vi "Teleop.vi"(10 "Match Info":T1={"Autonomous Elapsed Seconds"=0.0, "TeleOp Elapsed Seconds"=0.0, "Disabled Elapsed Seconds"=0.0, "Visited Autonomous"=FALSE, "Visited TeleOp"=FALSE, "Visited Disabled"=FALSE, "Autonomous Settings"={"Autonomous Style"=enum."Independent", "VI Refnum"=refnum}}, 11 "Call Context":T2) -> ()   [LabVIEW 2014]
doc: "This VI is called for each TeleOp packet received from the DS where the robot is not disabled. It is often used to read from the joysticks and update I/O or to update setpoints for timed control loops. It should complete and return within 20 milliseconds or it may miss DS packets."
uses:
  <vilib>/Rock Robotics/WPI/DriverStation/WPI_DriverStationDerivedRobotMode.ctl
  <vilib>/Rock Robotics/WPI/DriverStation/WPI_DriverStationMatch Info.ctl
  Drivetrain Code/Drivetrain Control.ctl
  Drivetrain Code/Drivetrain Mode.ctl
  Common Code/Solenoid Command.ctl
  <vilib>/Rock Robotics/WPI/Joystick/WPI_JoystickGetSetRefNum.vi
  <vilib>/Rock Robotics/Network Tables/SD Write Boolean Array.vi
  <vilib>/Rock Robotics/Network Tables/SD Write Numeric Array.vi
  Robot Global Data.vi
  <vilib>/Rock Robotics/Network Tables/SD Read Number.vi
  <vilib>/Rock Robotics/WPI/Solenoid/WPI_SolenoidSetEnum.vi
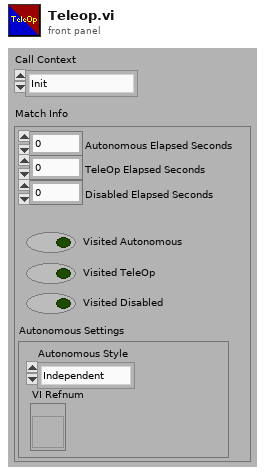
[diagram p1: front panel]
types:
  T1 = typedef "WPI_DriverStationMatch Info.ctl" = cluster{"Autonomous Elapsed Seconds":dbl, "TeleOp Elapsed Seconds":dbl, "Disabled Elapsed Seconds":dbl, "Visited Autonomous":bool, "Visited TeleOp":bool, "Visited Disabled":bool, "Autonomous Settings":cluster{"Autonomous Style":enum16{"Iterative", "Independent"}, "VI Refnum":refnum<vi>}}
  T2 = typedef "WPI_DriverStationDerivedRobotMode.ctl" = enum16{"Init", "Execute", "Stop"}
  T3 = typedef "Solenoid Command.ctl" = cluster{"Lift":bool, "Gripper":bool}
  T4 = typedef "Drivetrain Control.ctl" = cluster{"Mode":T5, "X":dbl, "Y":dbl, "Heading Target":dbl, "Y Target":dbl}
  T5 = typedef "Drivetrain Mode.ctl" = enum16{"Manual", "Gyro Steer", "Vision Steer", "Drive Distance"}
  T6 = typedef "WPI_JoystickDevRef.ctl" = cluster{"Device":T7}
  T7 = typedef "WPI_JoystickDeviceEnum.ctl" = enum16{"USB 0", "USB 1", "USB 2", "USB 3", "USB 4", "USB 5"}
  T8 = cluster{"Buttons[0]":bool, "Buttons[1]":bool, "Buttons[2]":bool, "Buttons[3]":bool, "Buttons[4]":bool, "Buttons[5]":bool, "Buttons[6]":bool, "Buttons[7]":bool, "Buttons[8]":bool}
  T9 = cluster{"Axes[0]":dbl, "Axes[1]":dbl, "Axes[2]":dbl, "Axes[3]":dbl, "Axes[4]":dbl, "Axes[5]":dbl, "Axes[6]":dbl, "Axes[7]":dbl, "Axes[8]":dbl}
  T10 = typedef "WPI_SolenoidDevRef.ctl" = cluster{"DevStatus":errorcluster, "Pneumatics Control Module":u8, "Forward Solenoid Channel":T11, "Reverse Solenoid Channel":T11}
  T11 = typedef "WPI_SolenoidChannel.ctl" = enum8{"Solenoid 0", "Solenoid 1", "Solenoid 2", "Solenoid 3", "Solenoid 4", "Solenoid 5", "Solenoid 6", "Solenoid 7", "Invalid"}
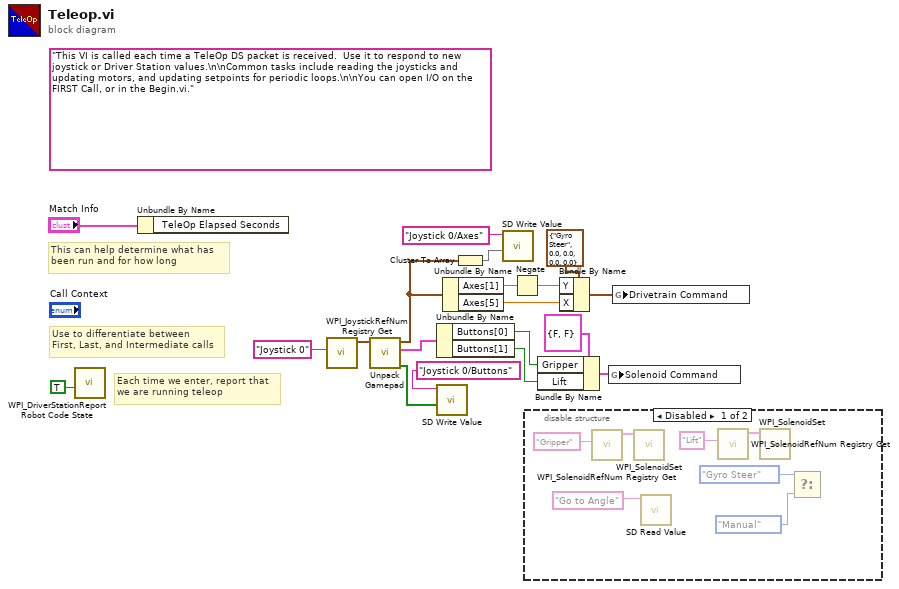
[diagram p0: block diagram]
diagram:
  (unwired) "This VI is called each time a TeleOp DS packet is received.  Use it to respond to new joystick or Driver Station values.\n\nCommon tasks include reading the joysticks and updating motors, and updating setpoints for periodic loops.\n\nYou can open I/O on the FIRST Call, or in the Begin.vi."
  # "Each time we enter, report that\nwe are running teleop"
  # "Use to differentiate between\nFirst, Last, and Intermediate calls"
  # "This can help determine what has\nbeen run and for how long"
  n1 = call <vilib>:"WPI_DriverStationReport Robot Code State.vi"("TeleOp"=TRUE ("Autonomous")) -> ()  [unwired: 10 in, 1 out]
  n2 = Unbundle By Name("Match Info") -> ()  [unwired: 1 out]
  n3 = call <vilib>:"WPI_JoystickRefNum Registry Get.vi"("refnum name"="Joystick 0") -> ("JoystickDevRef"=w14:T6)  [unwired: 1 in, 9 out]
  n4 = call "Unpack Gamepad.vi"("JoystickDevRef"=w14) -> ("Button Array"=w12:bool[], "Button Cluster"=w13:T8, "Axes"=w11:T9)  [unwired: 7 in, 1 out]
  n5 = Unbundle By Name(w13) -> ("Buttons[0]"=w2:bool, "Buttons[1]"=w3:bool)
  n6 = call-poly <vilib>:"SD Write Value.vi"("Boolean Array"=w12, "Name"="Joystick 0/Buttons") -> ()  [unwired: 8 in, 2 out]
  n7 = Unbundle By Name(w11) -> ("Axes[1]"=w5:dbl, "Axes[5]"=w9:dbl)
  n8 = Cluster To Array(cluster=w11) -> (array=w10:dbl[])
  n9 = call-poly <vilib>:"SD Write Value.vi"("Numeric Array"=w10, "Name"="Joystick 0/Axes") -> ()  [unwired: 8 in, 2 out]
  n10 = Negate(x=w5) -> (-x=w4:dbl)
  n11 = disable-structure shown="Disabled" {
    frame Disabled {
      n12 = call <vilib>:"WPI_SolenoidRefNum Registry Get.vi"("refnum name"="Gripper") -> ("SolenoidDevRef"=w23:T10)  [unwired: 9 in, 1 out]
      n13 = call-poly <vilib>:"WPI_SolenoidSet.vi"("SolenoidDevRef"=w23) -> ()  [unwired: 9 in, 2 out]
      n14 = call-poly <vilib>:"SD Read Value.vi"("Name"="Go to Angle") -> ()  [unwired: 8 in, 3 out]
      n15 = call <vilib>:"WPI_SolenoidRefNum Registry Get.vi"("refnum name"="Lift") -> ("SolenoidDevRef"=w26:T10)  [unwired: 9 in, 1 out]
      n16 = call-poly <vilib>:"WPI_SolenoidSet.vi"("SolenoidDevRef"=w26) -> ()  [unwired: 9 in, 2 out]
      n17 = Select(t=enum16{"Gyro Steer"}."Gyro Steer", f=enum16{"Manual", "Gyro Steer"}."Manual") -> ()  [unwired: 1 in, 1 out]
    }
    frame Enabled {
    }
  }
  n18 = Bundle By Name(cluster=T3 {"Lift"=FALSE, "Gripper"=FALSE} ("Solenoid Command"), "Gripper"=w2, "Lift"=w3) -> (w6:T3)
  n19 = Bundle By Name(cluster=T4 {"Mode"=enum."Gyro Steer", "X"=0.0, "Y"=0.0, "Heading Target"=0.0, "Y Target"=0.0} ("Drivetrain Command"), "Y"=w4, "X"=w9) -> (w1:T4)
  n20 = global write "Robot Global Data.vi" "Solenoid Command"(w6) -> ()
  n21 = global write "Robot Global Data.vi" "Drivetrain Command"(w1) -> ()
